vi "Write Loop Structure.vi"(8 "error in (no error)":errorcluster, 10 "Loop Structure":refnum<vi>, 11 "DMA Loop in":refnum<class "DMA Loop.lvclass">) -> (0 "error out":errorcluster, 3 "DMA Loop out":refnum<class "DMA Loop.lvclass">)   [LabVIEW 2015, in "DMA Loop.lvclass"]
uses:
  DMA Loop.lvclass
  DMA Loop.lvclass/DMA Loop.ctl
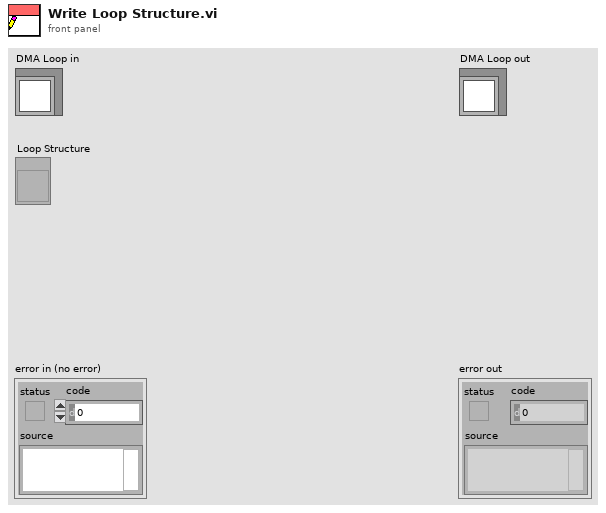
[diagram p1: front panel]
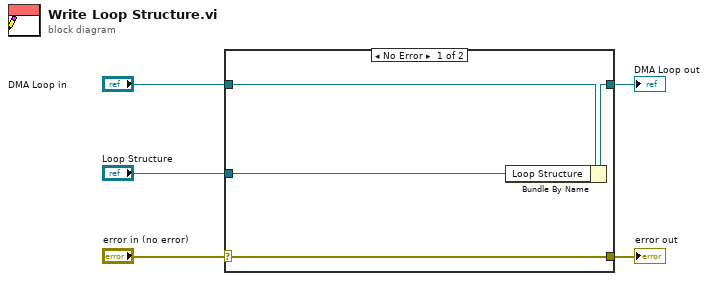
[diagram p0: block diagram]
diagram:
  n1 = case shown="No Error" "error in (no error)" {
    selector: "error in (no error)" -> [w9 w10]
    tunnel: [w9 w10] -> w4
    tunnel: [w7 w11] -> w2
    tunnel: "DMA Loop in" -> [w8 w11]
    tunnel: "Loop Structure" -> [w6 _]
    frame No Error {
      n2 = Bundle By Name(cluster=w8, "Loop Structure"=w6) -> (w7:refnum<class "DMA Loop.lvclass">)
    }
    frame Error {
    }
  }
  "error out" <- w4
  "DMA Loop out" <- w2
